vi "PE Create.vi"(8 "error in (no error)":errorcluster, 11 "conffile":string) -> (0 "error out":errorcluster, 2 "function return":i32, 3 "peHandle":u32)   [LabVIEW 2011, in "libPhyspec.lvlib"]
doc: "PHYSPEC_API PE_STATUS PE_Create(const char *conffile, PE_HANDLE *peHandle);"
uses:
  libPhyspec.lvlib
  libPhyspec.dll
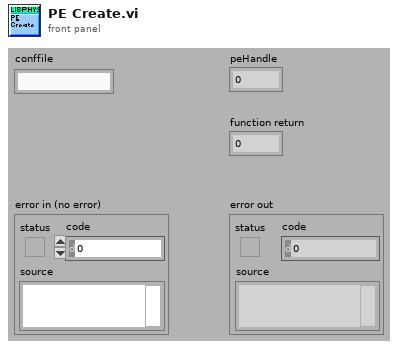
[diagram p1: front panel]
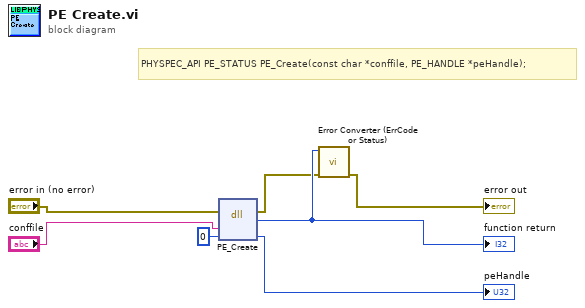
[diagram p0: block diagram]
diagram:
  # "PHYSPEC_API PE_STATUS PE_Create(const char *conffile, PE_HANDLE *peHandle);"
  n1 = dll-call lib="D:/users/nicolas/PHySpec-SDK-1.0.0/Labview-example/libPhyspec/libPhyspec.*" fn="PE_Create"(error in="error in (no error)", "conffile"="conffile", "peHandle"=u32 0) -> (error out=w2:errorcluster, w7:i32, "peHandle"=→"peHandle":u32)  [unwired: 3 in, 1 out]
  "function return" <- w7
  n2 = call "Error Converter (ErrCode or Status).vi"("error in (no error)"=w2, "error code"=w7) -> ("error out"=→"error out":errorcluster)  [unwired: 9 in]
